vi "DMM_Get Reference.vi"(8 "error in (no error)":errorcluster, 11 "Instrument Reference":u8) -> (0 "error out":errorcluster, 2 "Class Attributes":T1, 3 "DMM Virtual.lvclass":refnum<class "DMM Virtual.lvclass">)   [LabVIEW 2018, in "DMM Virtual.lvclass"]
uses:
  DMM Virtual.lvclass
  Controls/Class Attributes Cluster.ctl
  DMM_Global.vi
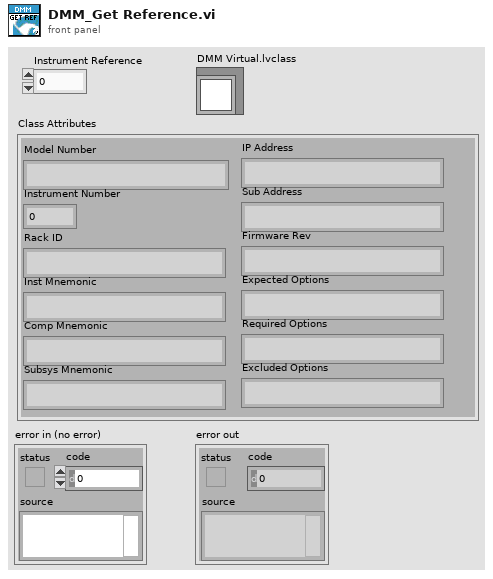
[diagram p1: front panel]
types:
  T1 = typedef "Class Attributes Cluster.ctl" = cluster{"Model Number":string, "Instrument Number":u8, "Rack ID":string, "Inst Mnemonic":string, "Comp Mnemonic":string, "Subsys Mnemonic":string, "IP Address":string, "Sub Address":string, "Firmware Rev":string, "Expected Options":string, "Required Options":string, "Excluded Options":string}
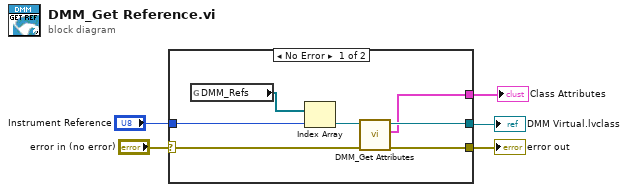
[diagram p0: block diagram]
diagram:
  n1 = case shown="No Error" "error in (no error)" {
    selector: "error in (no error)" -> [w10 w13]
    tunnel: [w9 w13] -> w4
    tunnel: "Instrument Reference" -> [w11 _]
    tunnel: [w7 _] -> w2
    tunnel: [w6 _] -> w1
    frame No Error {
      n2 = global read "DMM_Global.vi" "DMM_Refs"() -> (w12:refnum<class "DMM Virtual.lvclass">[])
      n3 = Index Array(array=w12, index=w11) -> (element=w8:refnum<class "DMM Virtual.lvclass">)
      n4 = call-dynamic "DMM_Get Attributes.vi"("error in (no error)"=w10, "DMM Virtual in"=w8) -> ("error out"=w9:errorcluster, "Class Attributes"=w6:T1, "DMM Virtual out"=w7:refnum<class "DMM Virtual.lvclass">)  [unwired: 7 in]
    }
    frame Error {
    }
  }
  "error out" <- w4
  "DMM Virtual.lvclass" <- w2
  "Class Attributes" <- w1
